vi "CaLabInfo.vi"() -> (0 "PV list":T1[](array[typedef]), 1 "EPICS environment":string[][](array[string]))   [LabVIEW 2022 SP3, in "CaLab.lvlib"]
doc: "This VI shows\n * EPICS environment variables\n * internal EPICS PV cache of CA Lab\n\nOUTPUT:\n <b>EPICS environment</b>\n currently used variables of EPICS environment\n <b>PV list</b>\n array of all EPICS PVs in the cache of CA Lab library"
uses:
  CaLab.lvlib
  <userlib>/calab/lib/calab.dll
  PV Info.ctl
panel:
  out "PVs":i32
  in  "Initialize (F)":bool
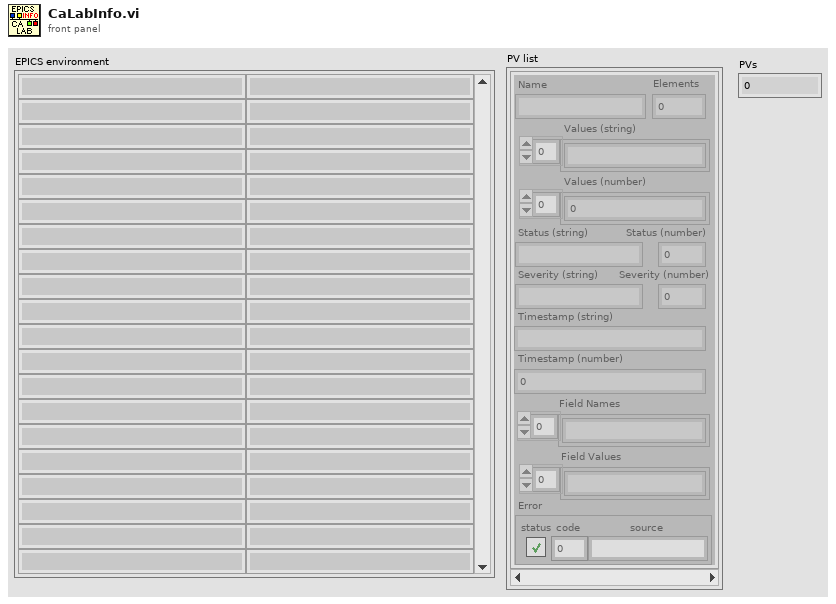
[diagram p1: front panel]
types:
  T1 = typedef "CaLab.lvlib/PV Info.ctl" = cluster{"Name":string, "Elements":i32, "Values (string)":string[], "Values (number)":dbl[], "Status (string)":string, "Status (number)":i16, "Severity (string)":string, "Severity (number)":i16, "Timestamp (string)":string, "Timestamp (number)":i32, "Field Names":string[], "Field Values":string[], "Error":errorcluster}
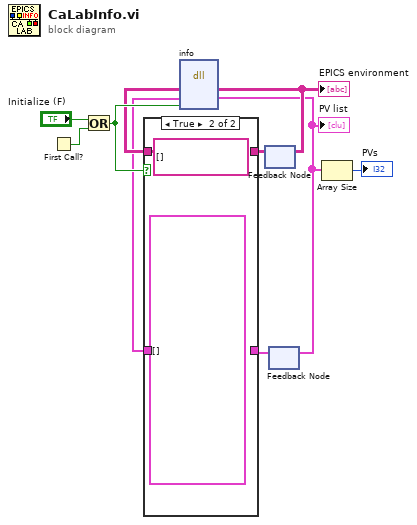
[diagram p0: block diagram]
diagram:
  n1 = First Call?() -> (First Call?: T/F=w9:bool)
  n2 = Or(x="Initialize (F)", y=w9) -> (x .or. y?=w8:bool)
  n3 = feedback #1() -> (w6:string[][])  [unwired: 1 out]
  n4 = feedback #2() -> (w3:T1[])  [unwired: 1 out]
  n5 = case shown="True" w8 {
    tunnel: w6 -> [w12 _]
    tunnel: [w12 string[][] [] ("CaLabInfo 2")] -> w5
    tunnel: [w11 T1[] [] ("PV Info")] -> w4
    tunnel: w3 -> [w11 _]
    frame False {
    }
    frame True {
    }
  }
  n6 = dll-call lib="C:/Program Files/National Instruments/LabVIEW 2023/user.lib/calab/lib/calab.dll" fn="info" label="caLabInfo"("InfoStringArray"=w5, "ArraySize"=w4, "FirstCall"=w8) -> ("InfoStringArray"=w7:string[][], "ArraySize"=w2:T1[])  [unwired: 4 in, 3 out]
  "EPICS environment" <- w7
  "PV list" <- w2
  n7 = feedback-in #1(w7) -> ()
  n8 = feedback-in #2(w2) -> ()
  n9 = Array Size(array=w2) -> (size(s)=→"PVs":i32)
